vi "matlab code in labview finding variable x.vi"() -> ()   [LabVIEW 2024]
panel:
  out "output variable 2":dbl
  out "output variable":dbl
  in  "input variable 3":dbl
  in  "input variable 2":dbl
  in  "input variable":dbl
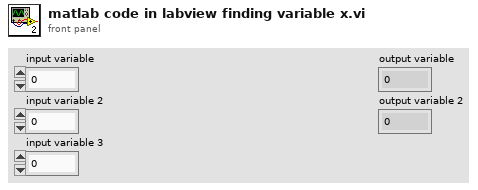
[diagram p1: front panel]
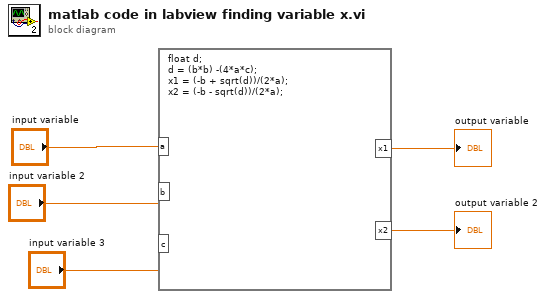
[diagram p0: block diagram]
diagram:
  n1 = formula code="float d;\nd = (b*b) -(4*a*c);\nx1 = (-b + sqrt(d))/(2*a);\nx2 = (-b - sqrt(d))/(2*a);"("a"="input variable", "b"="input variable 2", "c"="input variable 3") -> ("x1"=→"output variable":dbl, "x2"=→"output variable 2":dbl)
